vi "equals.vi"(8 "error in (no error)":errorcluster, 10 "object 2":refnum<class>, 11 "pShape in":refnum<class "pShape.lvclass">) -> (0 "error out":errorcluster, 2 "equal?":bool, 3 "pShape out":refnum<class "pShape.lvclass">)   [LabVIEW 2017, in "pShape.lvclass"]
uses:
  pShape.lvclass
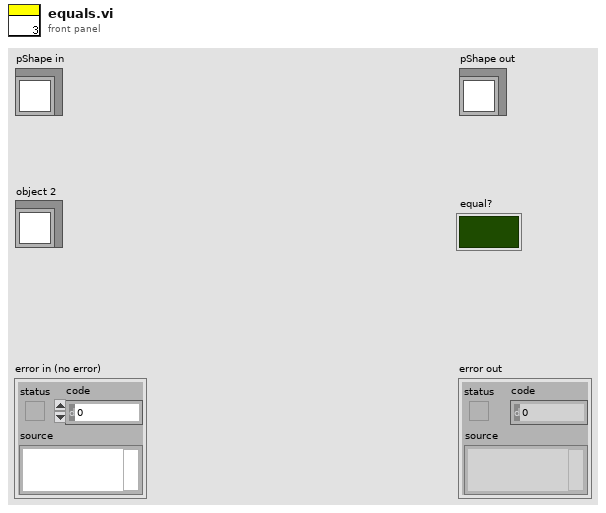
[diagram p1: front panel]
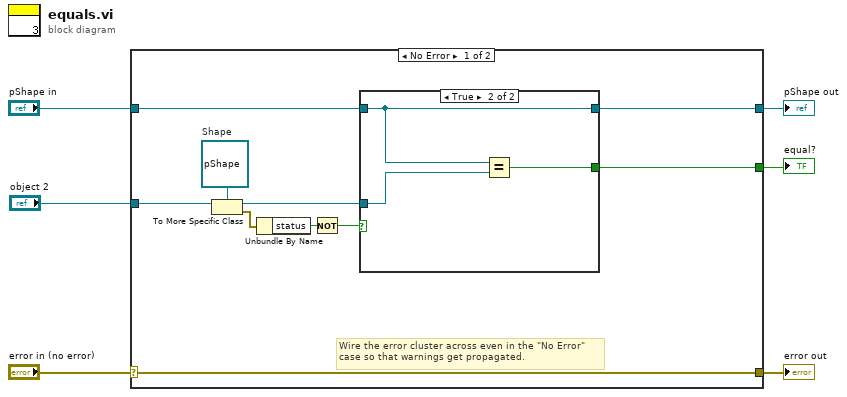
[diagram p0: block diagram]
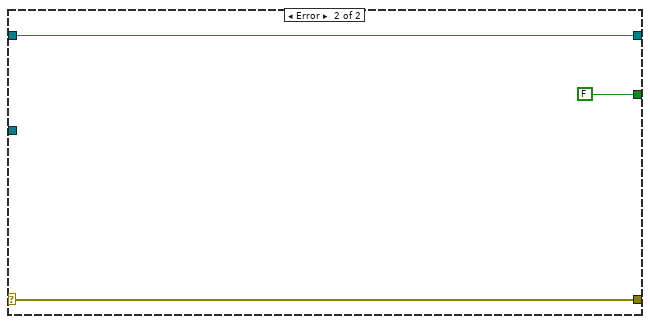
[diagram p3: hidden frame]
diagram:
  n1 = case shown="No Error" "error in (no error)" {
    selector: "error in (no error)" -> [w16 w24]
    tunnel: [w16 w24] -> w5
    tunnel: [w10 w23] -> w3
    tunnel: "pShape in" -> [w13 w23]
    tunnel: "object 2" -> [w15 _]
    tunnel: [w8 FALSE] -> w1
    frame No Error {
      w14 = refnum<class "pShape.lvclass"> refnum  # Shape
      # "Wire the error cluster across even in the \"No Error\"\ncase so that warnings get propagated."
      n2 = To More Specific Class(target class=w14, reference=w15) -> (specific class reference=w12:refnum<class "pShape.lvclass">, error out=w11:errorcluster)  [unwired: 1 in]
      n3 = Unbundle By Name(w11) -> ("status"=w9:bool)
      n4 = Not(x=w9) -> (.not. x?=w7:bool)
      n5 = case shown="True" w7 {
        selector: w7 -> [w17 _]
        tunnel: w13 -> [w18 w20]
        tunnel: w12 -> [_ w21]
        tunnel: [w18 w20] -> w10
        tunnel: [w17 w19] -> w8
        frame False {
        }
        frame True {
          n6 = Equal?(x=w20, y=w21) -> (x = y?=w19:bool)
        }
      }
    }
    frame Error {
    }
  }
  "error out" <- w5
  "pShape out" <- w3
  "equal?" <- w1
